vi "readFromXML.vi"(8 "error in (no error)":errorcluster, 10 "XML in":string, 11 "SetAccessMode in":refnum<class "SetAccessMode.lvclass">) -> (0 "error out":errorcluster, 3 "SetAccessMode out":refnum<class "SetAccessMode.lvclass">)   [LabVIEW 2022 SP3, in "TCSDataDefinitions.lvlib" / "TCSCommand.lvlib" / "SetAccessMode.lvlib" / "SetAccessMode.lvclass"]
uses:
  SetAccessMode.lvclass
  TCSTcsCommand/TCSTcsCommand.lvclass
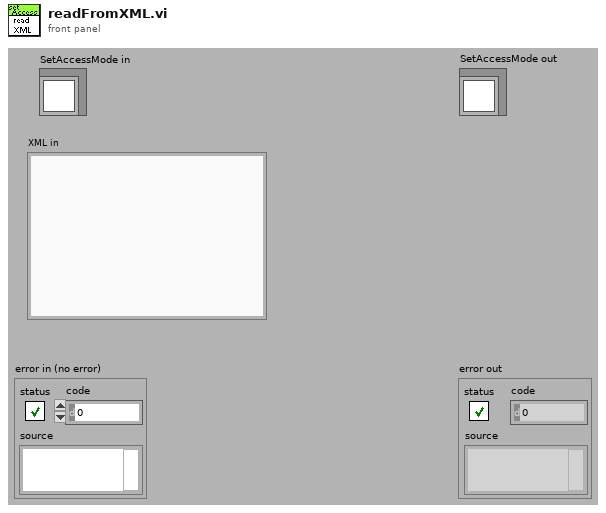
[diagram p1: front panel]
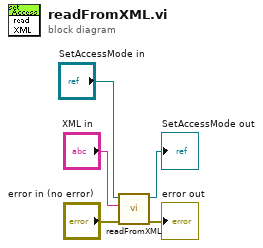
[diagram p0: block diagram]
diagram:
  n1 = call-parent "readFromXML.vi"("error in (no error)"="error in (no error)", "XMLin"="XML in", "TCSTcsCommand in"="SetAccessMode in") -> ("error out"=→"error out":errorcluster, "TCSTcsCommand out"=→"SetAccessMode out":refnum<class "SetAccessMode.lvclass">)  [unwired: 7 out]
